vi "events-init.vi"(0 "error out":errorcluster, 5 "entrée d'erreur (pas d'erreur)":errorcluster) -> (8 "Update graphs of exp":refnum<user-event>, 9 "Refnum d'abonnement à des événements 2":refnum<event-registration>, 10 "Measure event":refnum<user-event>, 11 "notifier out 2":refnum<notifier>, 12 "Refnum d'abonnement à des événements":refnum<event-registration>, 13 "notifier out":refnum<notifier>, 14 "Événement utilisateur en sortie":refnum<user-event>, 15 "Reglage event":refnum<user-event>, 16 "Refnum d'abonnement à des événements 3":refnum<event-registration>, 17 "Stop event":refnum<user-event>, 18 "Measure finished":refnum<user-event>, 19 "sortie d'erreur":errorcluster)   [LabVIEW 2015]
uses:
  Classes/Experiment.lvclass
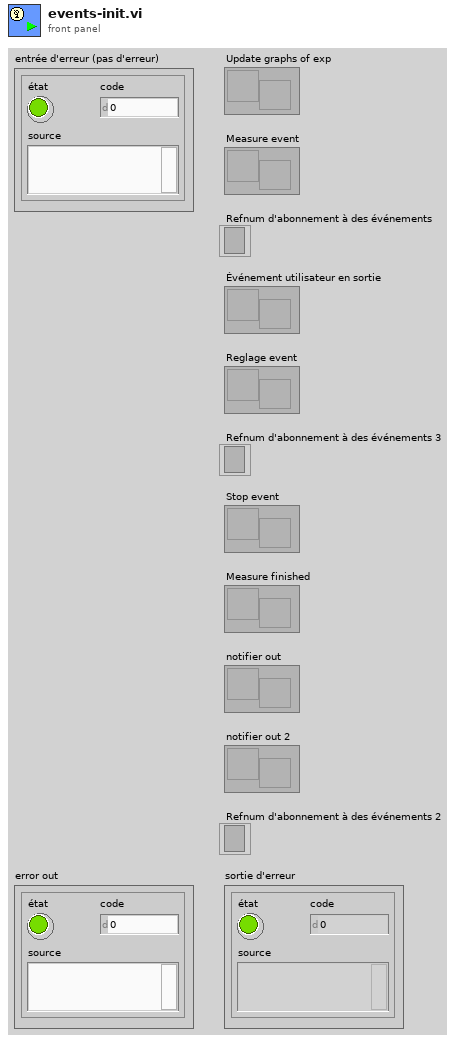
[diagram p1: front panel]
types:
  T1 = cluster{"Operate":bool, "Experiment":refnum<class "Experiment.lvclass">, "group path":path}
  T2 = cluster{"Operate":bool, "Experiment":refnum<class "Experiment.lvclass">}
  T3 = cluster{"Full/Part":bool, "Item names":string[], "Exp number":i32}
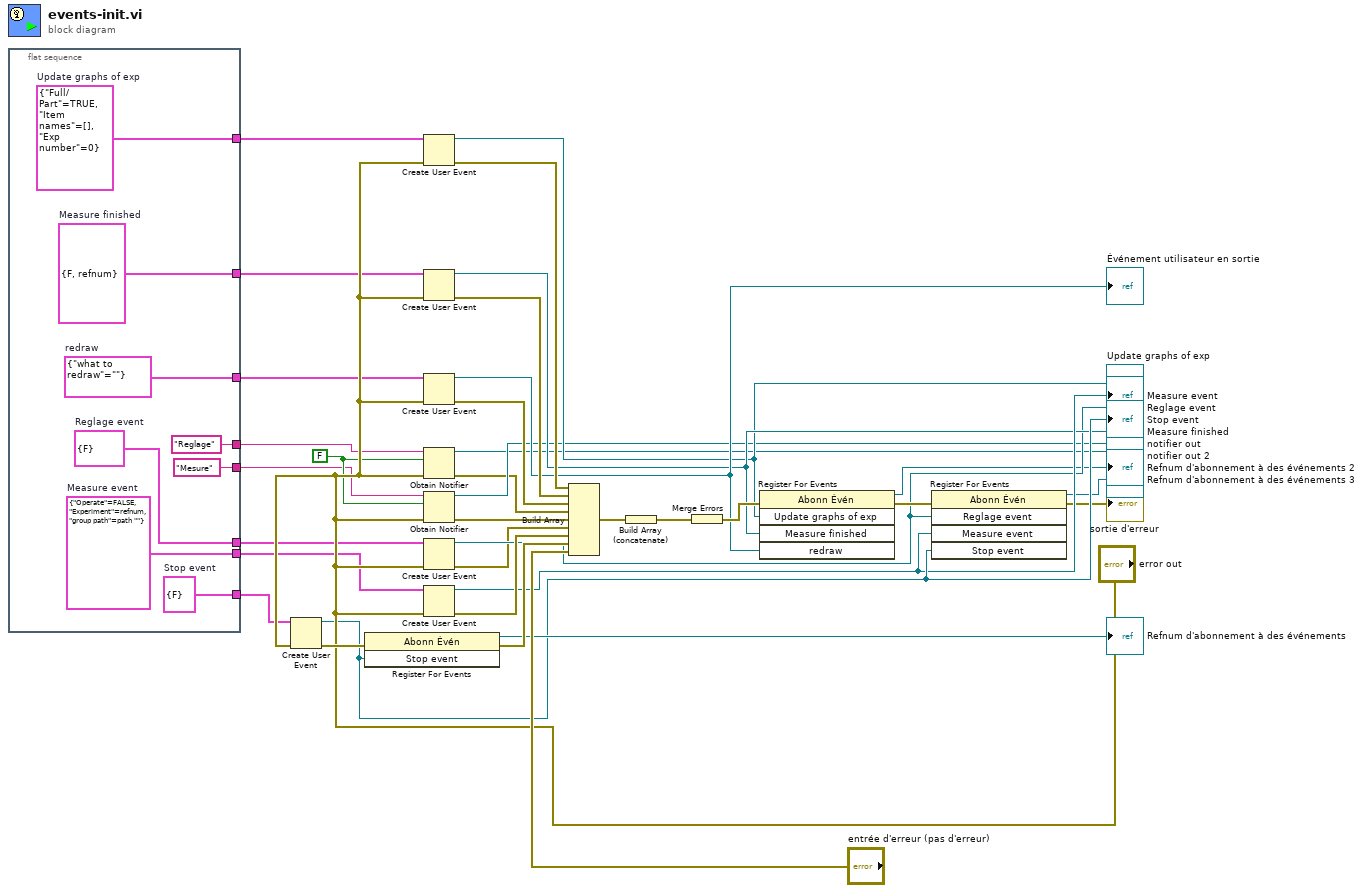
[diagram p0: block diagram]
diagram:
  w16 = FALSE
  n1 = flat-sequence {
    tunnel: [w44] -> w1
    tunnel: [w43] -> w2
    tunnel: [w42] -> w3
    tunnel: ["Mesure" ("name (unnamed)")] -> w4
    tunnel: ["Reglage" ("name (unnamed)")] -> w5
    tunnel: [w39] -> w17
    tunnel: [w38] -> w19
    tunnel: [w37] -> w21
    frame #0 {
      w37 = T1 {"Operate"=FALSE, "Experiment"=refnum, "group path"=path ""}  # Measure event
      w38 = cluster{"what to redraw":string} {"what to redraw"=""}  # redraw
      w39 = T2 {"Operate"=FALSE, "Experiment"=refnum}  # Measure finished
      w43 = cluster{"Stop":bool} {"Stop"=FALSE}  # Stop event
      w44 = T3 {"Full/Part"=TRUE, "Item names"=[], "Exp number"=0}  # Update graphs of exp
      w42 = cluster{"Operate":bool} {"Operate"=FALSE}  # Reglage event
    }
  }
  n2 = Create User Event(user event datatype=w2, error in="error out") -> (user event=w26:refnum<user-event>, error out=w34:errorcluster)
  "Stop event" <- w26
  n3 = register-events(error in=w34, w26) -> (reference out=→"Refnum d'abonnement à des événements":refnum<event-registration>, error out=w35:errorcluster)  [unwired: 1 in]
  n4 = Create User Event(user event datatype=w1, error in="error out") -> (user event=w14:refnum<user-event>, error out=w28:errorcluster)
  "Update graphs of exp" <- w14
  n5 = Create User Event(user event datatype=w17, error in="error out") -> (user event=w18:refnum<user-event>, error out=w29:errorcluster)
  "Measure finished" <- w18
  n6 = Create User Event(user event datatype=w19, error in="error out") -> (user event=w20:refnum<user-event>, error out=w30:errorcluster)
  "Événement utilisateur en sortie" <- w20
  n7 = Obtain Notifier(name (unnamed)=w5, notification data type=w16, error in (no error)="error out") -> (notifier out=→"notifier out 2":refnum<notifier>, error out=w7:errorcluster)  [unwired: 1 in, 1 out]
  n8 = Obtain Notifier(name (unnamed)=w4, notification data type=w16, error in (no error)="error out") -> (notifier out=→"notifier out":refnum<notifier>, error out=w8:errorcluster)  [unwired: 1 in, 1 out]
  n9 = Create User Event(user event datatype=w3, error in="error out") -> (user event=w15:refnum<user-event>, error out=w6:errorcluster)
  "Reglage event" <- w15
  n10 = Create User Event(user event datatype=w21, error in="error out") -> (user event=w22:refnum<user-event>, error out=w23:errorcluster)
  "Measure event" <- w22
  n11 = Build Array(w28, w29, w30, w7, w8, w6, w23, w35, "entrée d'erreur (pas d'erreur)") -> (w24:errorcluster[])
  n12 = Build Array (concatenate)(w24) -> (w25:errorcluster[])
  n13 = Merge Errors(w25) -> (w31:errorcluster)
  n14 = register-events(error in=w31, w14, w18, w20) -> (reference out=→"Refnum d'abonnement à des événements 2":refnum<event-registration>, error out=w32:errorcluster)  [unwired: 1 in]
  n15 = register-events(error in=w32, w15, w22, w26) -> (reference out=→"Refnum d'abonnement à des événements 3":refnum<event-registration>, error out=→"sortie d'erreur":errorcluster)  [unwired: 1 in]
